vi "Add Handler.vi"(8 "error in":errorcluster, 10 "Handler":refnum<class "Handler.lvclass">, 11 "Logger in":refnum<class "Logger.lvclass">) -> (0 "error out":errorcluster, 3 "Logger out":refnum<class "Logger.lvclass">)   [LabVIEW 2020, in "hse-logger.lvlib" / "Logger.lvclass"]
doc: "Adds a ``Handler`` to this Logger.\n\n____\nHAMPEL SOFTWARE ENGINEERING v2.0.6 (2021-04-15 11:38)"
uses:
  Logger.lvclass
  Handler/Handler.lvclass
  Logger.lvclass/Logger.ctl
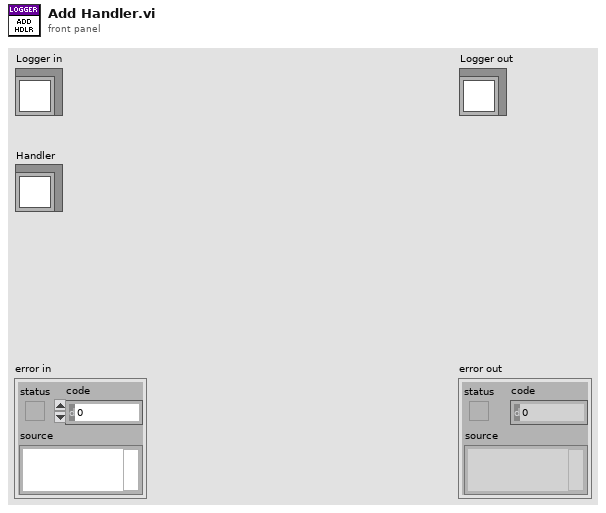
[diagram p1: front panel]
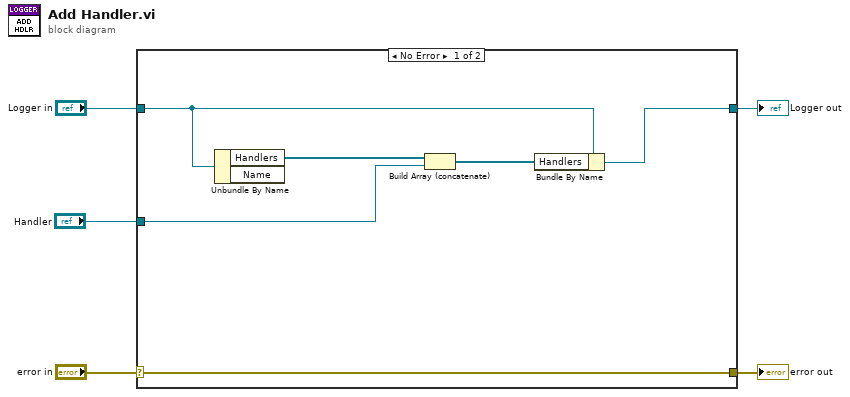
[diagram p0: block diagram]
diagram:
  n1 = case shown="No Error" "error in" {
    selector: "error in" -> [w6 w13]
    tunnel: [w6 w13] -> w4
    tunnel: [w8 w12] -> w2
    tunnel: "Logger in" -> [w9 w12]
    tunnel: "Handler" -> [w10 _]
    frame No Error {
      n2 = Unbundle By Name(w9) -> ("Handlers"=w11:refnum<class "Handler.lvclass">[])  [unwired: 1 out]
      n3 = Build Array (concatenate)(w11, w10) -> (w7:refnum<class "Handler.lvclass">[])
      n4 = Bundle By Name(cluster=w9, "Handlers"=w7) -> (w8:refnum<class "Logger.lvclass">)
    }
    frame Error {
    }
  }
  "error out" <- w4
  "Logger out" <- w2
